vi "Get.vi"(11 "Created Info in":refnum<class "Created Info.lvclass">) -> (0 "Actor":refnum<class "Actor.lvclass">, 1 "Is Normal":bool, 2 "Created Attributes":T1)   [LabVIEW 2021, in "jettl.lvlib" / "Actor.lvlib" / "Created Info.lvclass"]
uses:
  Created Info.lvclass
  Attributes.ctl
  Msg/Msg.lvclass
  Implemented Msgs.ctl
  Actor/Actor.lvclass
  Created Info.lvclass/Created Info.ctl
  Actor.lvlib
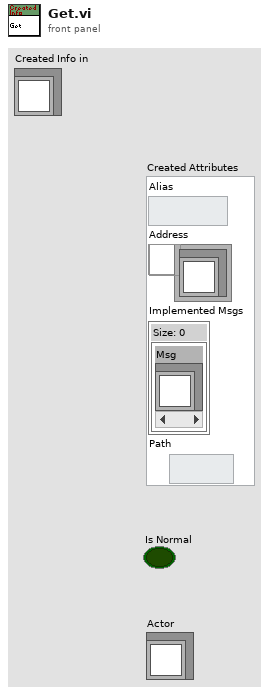
[diagram p1: front panel]
types:
  T1 = typedef "jettl.lvlib/Actor.lvlib/Attributes.ctl" = cluster{"Alias":string, "Address":refnum<user-event>, "Implemented Msgs":T2, "Path":path}
  T2 = typedef "jettl.lvlib/Actor.lvlib/Implemented Msgs.ctl" = set{refnum<class "Msg.lvclass">}
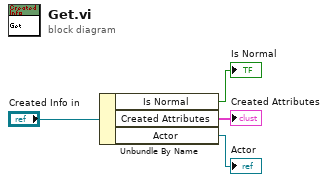
[diagram p0: block diagram]
diagram:
  n1 = Unbundle By Name("Created Info in") -> ("Is Normal"=→"Is Normal":bool, "Created Attributes"=→"Created Attributes":T1, "Actor"=→"Actor":refnum<class "Actor.lvclass">)
